vi "VI Tools.vi"() -> ()   [LabVIEW 2020]
panel:
  in  "确定":bool
  out "进度条":u64(slide) scale=0.0..10.0
  in  "LabView 版本":string(combo)="20.0"
  in  "Folder Path":path caption="文件夹路径"
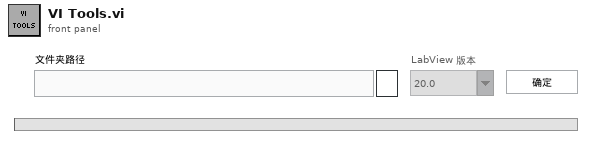
[diagram p1: front panel]
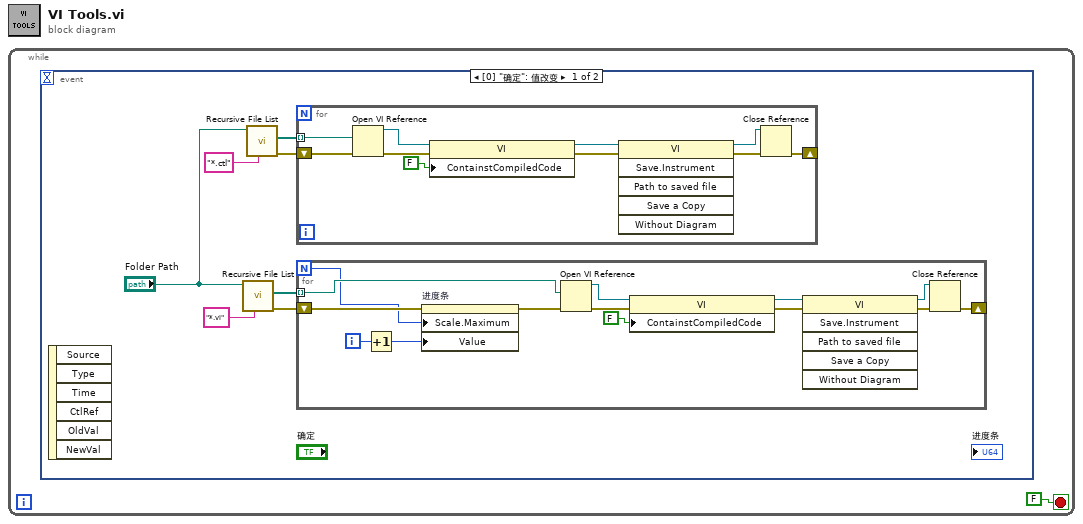
[diagram p0: block diagram]
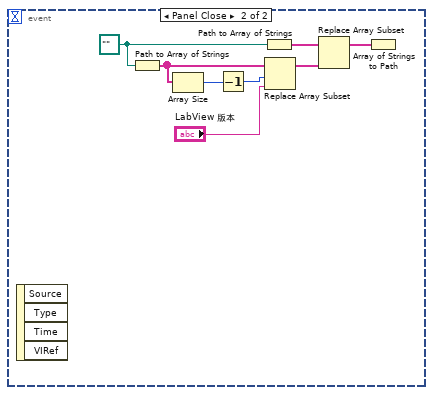
[diagram p2: hidden frame]
diagram:
  n1 = while {
    stop <- FALSE stop-if-true
    n2 = event shown="[0] \"确定\": 值改变" {
      selector: _ -> [_ _]
      dyn-events: _ -> [_ _]
      timeout: _ -> [_ _]
      event "确定": Value Change {
        n3 = event-data() -> ()  [unwired: 1 in, 6 out]
        n4 = call <vilib>:"Recursive File List.vi"("pattern"="*.vi", "Folder Path"="Folder Path") -> ("error out"=w4:errorcluster, "All Files in Dir"=w8:path[])  [unwired: 5 in, 3 out]
        n5 = call <vilib>:"Recursive File List.vi"("pattern"="*.ctl", "Folder Path"="Folder Path") -> ("error out"=w3:errorcluster, "All Files in Dir"=w5:path[])  [unwired: 5 in, 3 out]
        n6 = for {
          tunnel: w5 -> [w9] mode=indexing
          shift-right: [w14] -> _
          shift-left: w3 -> [w13]
          n7 = Open VI Reference(vi path=w9, error in (no error)=w13) -> (vi reference=w18:refnum<vi>, error out=w12:errorcluster)  [unwired: 4 in]
          n8 = property class="VI"(reference=w18, error in=w12, "ContainstCompiledCode"=FALSE ("包含已编译代码")) -> (reference out=w17:refnum<vi>, error out=w11:errorcluster)
          n9 = invoke class="VI" method="Save.Instrument"(reference=w17, error in=w11) -> (reference out=w15:refnum<vi>, error out=w10:errorcluster)  [unwired: 4 in, 4 out]
          n10 = Close Reference(reference=w15, error in (no error)=w10) -> (error out=w14:errorcluster)
        }
        n11 = for {
          N -> [w20]
          tunnel: w8 -> [w24] mode=indexing
          shift-right: [w28] -> _
          shift-left: w4 -> [w22]
          i -> [w23]
          n12 = Increment(x=w23) -> (x+1=w19:i32)
          n13 = property on="进度条" class="Slide (严格)"(error in=w22, "Scale.Maximum"=w20, "Value"=w19) -> (error out=w21:errorcluster)  [unwired: 1 in, 1 out]
          n14 = Open VI Reference(vi path=w24, error in (no error)=w21) -> (vi reference=w32:refnum<vi>, error out=w27:errorcluster)  [unwired: 4 in]
          n15 = property class="VI"(reference=w32, error in=w27, "ContainstCompiledCode"=FALSE ("包含已编译代码")) -> (reference out=w31:refnum<vi>, error out=w26:errorcluster)
          n16 = invoke class="VI" method="Save.Instrument"(reference=w31, error in=w26) -> (reference out=w29:refnum<vi>, error out=w25:errorcluster)  [unwired: 4 in, 4 out]
          n17 = Close Reference(reference=w29, error in (no error)=w25) -> (error out=w28:errorcluster)
        }
      }
      event Panel Close {
        w33 = path "" ("Folder Path")
        n18 = event-data() -> ()  [unwired: 1 in, 4 out]
        n19 = Path to Array of Strings(0:w33) -> (2:w39:string[])  [unwired: 1 out]
        n20 = Array Size(array=w39) -> (size(s)=w38:i32)
        n21 = Decrement(x=w38) -> (x-1=w37:i32)
        n22 = Path to Array of Strings(0:w33) -> (2:w35:string[])  [unwired: 1 out]
        n23 = Replace Array Subset(array=w39, new element="LabView 版本", index=w37) -> (w34:string[])
        n24 = Replace Array Subset(array=w35, new element=w34) -> (w36:string[])  [unwired: 1 in]
        n25 = Array of Strings to Path(0:w36) -> ()  [unwired: 1 in, 1 out]
      }
    }
  }
